vi "Update_Holo_Array_SLM.vi"(8 "Holo Array In":T1[](array[typedef]) {"Modes"."Amplititute" step=0.05}, 9 "Holo ID":i32, 10 "Mode ID":i32, 11 "Amplititute":dbl) -> (0 "Update Holo Array":T1[](array[typedef]) {"Modes"."Amplititute" step=0.05})   [LabVIEW 2014]
uses:
  Controls/Holo Settings.ctl
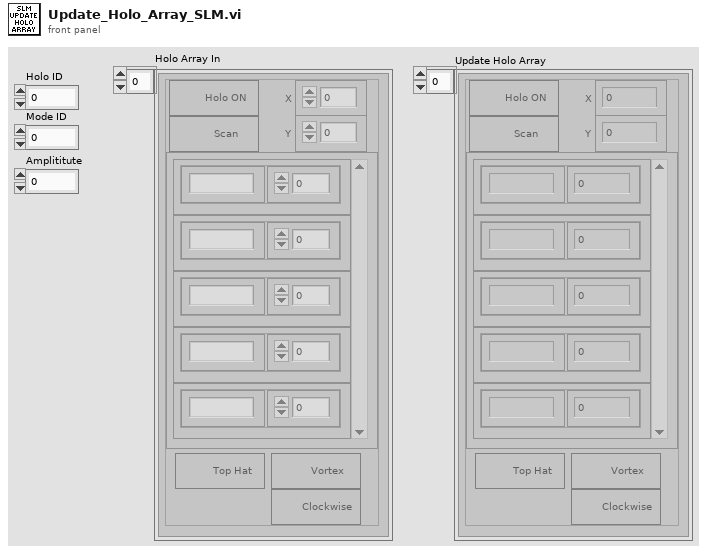
[diagram p1: front panel]
types:
  T1 = typedef "Holo Settings.ctl" = cluster{"Top Hat":bool, "Modes":cluster{"Mode ID":string, "Amplititute":dbl}[], "Vortex":bool, "Clockwise":bool, "X":dbl, "Y":dbl, "Holo ON":bool, "Scan":bool}
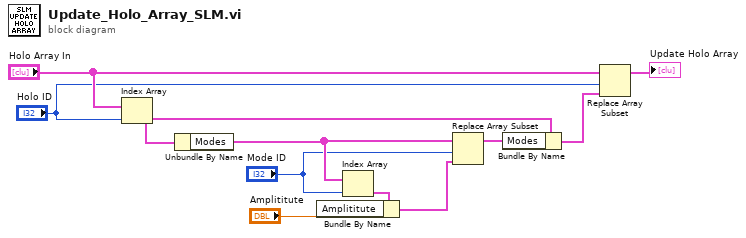
[diagram p0: block diagram]
diagram:
  n1 = Index Array(array="Holo Array In", index="Holo ID") -> (element=w6:T1)
  n2 = Unbundle By Name(w6) -> ("Modes"=w9:cluster{"Mode ID":string, "Amplititute":dbl}[])
  n3 = Index Array(array=w9, index="Mode ID") -> (element=w11:cluster{"Mode ID":string, "Amplititute":dbl})
  n4 = Bundle By Name(cluster=w11, "Amplititute"="Amplititute") -> (w8:cluster{"Mode ID":string, "Amplititute":dbl})
  n5 = Replace Array Subset(array=w9, new element=w8, index="Mode ID") -> (w5:cluster{"Mode ID":string, "Amplititute":dbl}[])
  n6 = Bundle By Name(cluster=w6, "Modes"=w5) -> (w3:T1)
  n7 = Replace Array Subset(array="Holo Array In", new element=w3, index="Holo ID") -> (→"Update Holo Array":T1[])
